vi "A33ConfigurePRBS.vi"(6 "Edge (4ns)":dbl=4e-09 format="%#_12g", 8 "error in (no error)":errorcluster, 9 "Sequenc type PN#":u16=7 min=3 max=32, 10 "Channel (1: Channel1)":u16(ring)=1 items=["Channel1"=1, "Channel2"=2], 11 "VISA resource name":refnum<visa-resource-name>) -> (0 "error out":errorcluster, 3 "VISA resource name out":refnum<visa-resource-name>)   [LabVIEW 2022 SP3]
doc: "Selects the waveform shape, frequency, amplitude, offset, and phase for a standard waveform."
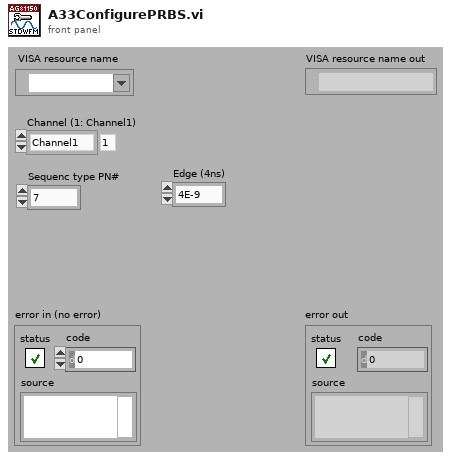
[diagram p1: front panel]
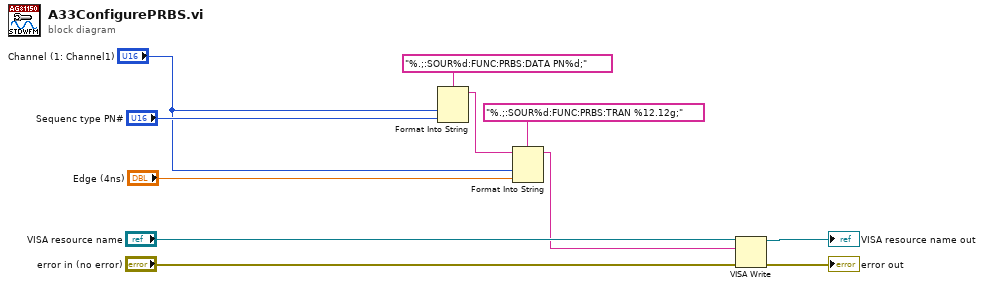
[diagram p0: block diagram]
diagram:
  n1 = Format Into String(format string="%.;:SOUR%d:FUNC:PRBS:DATA PN%d;", "Channel (1: Channel1)", "Sequenc type PN#") -> (resulting string=w8:string)  [unwired: 2 in, 1 out]
  n2 = Format Into String(format string="%.;:SOUR%d:FUNC:PRBS:TRAN %12.12g;", initial string=w8, "Channel (1: Channel1)", "Edge (4ns)") -> (resulting string=w1:string)  [unwired: 1 in, 1 out]
  n3 = VISA Write(VISA resource name="VISA resource name", write buffer=w1, error in (no error)="error in (no error)") -> (VISA resource name out=→"VISA resource name out":refnum<visa-resource-name>, error out=→"error out":errorcluster)  [unwired: 1 out]
